vi "loadChannelArray.vi"(6 "type":string, 8 "error in (no error)":errorcluster, 9 "device.lvclass":refnum<class "device.lvclass">, 10 "NativeXML in":refnum<class "NativeXML.lvclass">, 11 "deviceDataBase in":refnum<class "deviceDataBase.lvclass">) -> (0 "error out":errorcluster, 1 "device.lvclass out":refnum<class "device.lvclass">, 2 "NativeXML out":refnum<class "NativeXML.lvclass">, 3 "deviceDataBase out":refnum<class "deviceDataBase.lvclass">)   [LabVIEW 2009, in "Tools.lvlib" / "DatabaseHelpers.lvlib" / "deviceDataBase.lvclass"]
uses:
  deviceDataBase.lvclass
  NativeXML/NativeXML.lvclass
  Database Objects/device/device.lvclass
  Database Objects/ChannelArray/ChannelArray.lvclass
panel:
  out "Numeric":i32
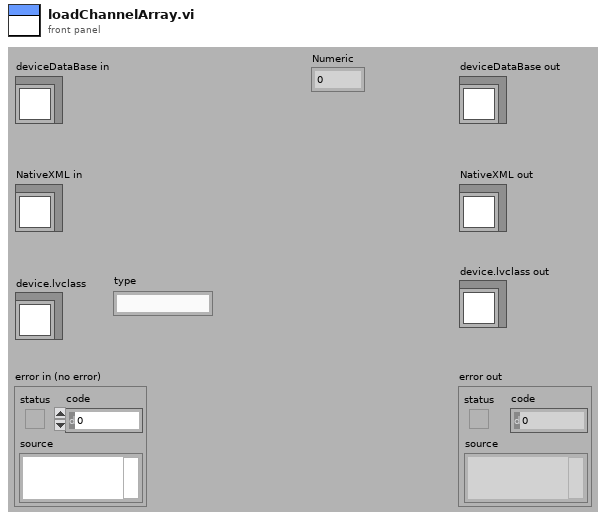
[diagram p1: front panel]
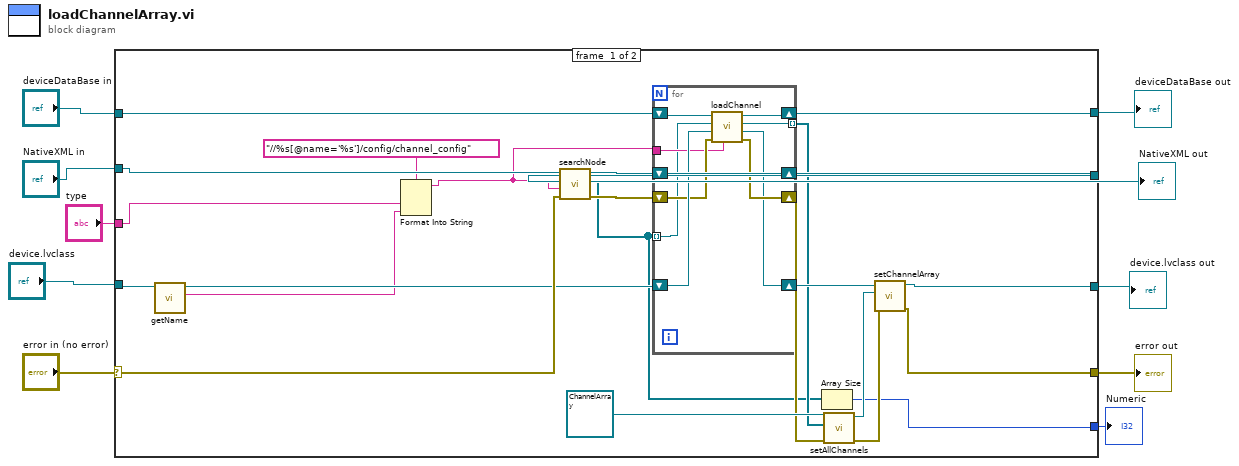
[diagram p0: block diagram]
diagram:
  n1 = case shown="No Error" "error in (no error)" {
    selector: "error in (no error)" -> [w23 w45]
    tunnel: [w26 w45] -> w9
    tunnel: [w32 w44] -> w7
    tunnel: "deviceDataBase in" -> [w33 w44]
    tunnel: "NativeXML in" -> [w20 _]
    tunnel: "device.lvclass" -> [w16 _]
    tunnel: [w31 _] -> w4
    tunnel: [w24 _] -> w3
    tunnel: [w18 _] -> w2
    tunnel: "type" -> [w17 _]
    frame #0 {
      n2 = call "getName.vi"("device.lvclass in"=w16) -> ("name"=w14:string, "device.lvclass out"=w15:refnum<class "device.lvclass">)  [unwired: 8 in, 1 out]
      n3 = Format Into String(format string="//%s[@name='%s']/config/channel_config", w17, w14) -> (resulting string=w11:string)  [unwired: 2 in, 1 out]
      n4 = call "searchNode.vi"("error in (no error)"=w23, "searchXPath"=w11, "NativeXML in"=w20) -> ("error out"=w22:errorcluster, "nodeArray"=w12:refnum<class "NativeXML.lvclass">[], "NativeXML out"=w21:refnum<class "NativeXML.lvclass">)  [unwired: 6 in]
      n5 = for {
        shift-right: [w41] -> w32
        shift-left: w33 -> [w42]
        shift-right: [w43] -> w31
        shift-left: w21 -> [w43]
        tunnel: w12 -> [w34] mode=indexing
        shift-right: [w37] -> w29
        shift-left: w15 -> [w40]
        shift-right: [w39] -> w28
        shift-left: w22 -> [w38]
        tunnel: [w36] -> w19 mode=indexing
        tunnel: w11 -> [w35]
        n6 = call "loadChannel.vi"("xmlPath"=w35, "error in (no error)"=w38, "device.lvclass"=w40, "NativeXML in"=w34, "deviceDataBase in"=w42) -> ("error out"=w39:errorcluster, "device.lvclass out"=w37:refnum<class "device.lvclass">, "Channel.lvclass"=w36:refnum<class "Channel.lvclass">, "deviceDataBase out"=w41:refnum<class "deviceDataBase.lvclass">)  [unwired: 3 in]
      }
      n7 = Array Size(array=w12) -> (size(s)=w18:i32)
      n8 = call "setAllChannels.vi"("error in (no error)"=w28, "channels"=w19, "ChannelArray.lvclass in"=refnum<class "ChannelArray.lvclass"> refnum ("Tools.lvlib:DatabaseHelpers.lvlib:ChannelArray.lvclass")) -> ("error out"=w27:errorcluster, "ChannelArray.lvclass out"=w25:refnum<class "ChannelArray.lvclass">)  [unwired: 7 in]
      n9 = call "setChannelArray.vi"("error in (no error)"=w27, "ChannelArray.lvclass"=w25, "device.lvclass in"=w29) -> ("error out"=w26:errorcluster, "device.lvclass out"=w24:refnum<class "device.lvclass">)  [unwired: 7 in]
    }
    frame #1 {
    }
  }
  "error out" <- w9
  "deviceDataBase out" <- w7
  "NativeXML out" <- w4
  "device.lvclass out" <- w3
  "Numeric" <- w2
